vi "Gets_data.vi"(0 "object in":refnum<class "212format_work.lvclass">, 5 "error in (no error)":errorcluster) -> (14 "object out":refnum<class "212format_work.lvclass">, 15 "data":T1={"选择发送的参数"="", "插值后的数组元素"={"PH"=[], "CODCr"=[], "氨氮"=[], "CODMn"=[], "总氮"=[], "总磷"=[], "电导率"=[], "水温"=[], "DO"=[], "浊度"=[], "叶绿素"=[], "藻密度"=[], "铜"=[], "盐度"=[], "水位"=[], "流速"=[], "瞬时流量"=[], "累积流量"=[], "亚硝酸盐"=[], "硫化物"=[], "ORP"=[], "铅"=[], "镉"=[], "锌"=[], "镍"=[], "锰"=[], "汞"=[], "气温"=[], "气压"=[], "风速"=[], "风向"=[], "盐度 2"=[], "磷酸盐"=[], "硝氮"=[], "氟化物"=[], "挥发酚"=[], "氯化物"=[]}, "register values"=[], "columns输出"=[], "环境参数"=[], "仪器编码"="", "实时数据发送间隔"=0, "实时数据参数"="水样测试", "参数系数簇"={"CODMn"=0.0, "CODCr"=0.0, "DO"=0.0, "铜"=0.0, "PH"=0.0, "氨氮"=0.0, "比电导率"=0.0, "水温"=0.0, "COD"=0.0, "浊度"=0.0, "总氮"=0.0, "总磷"=0.0, "叶绿素a"=0.0, "藻密度"=0.0, "水位"=0.0, "流速"=0.0, "瞬时流量"=0.0, "累积流量"=0.0, "亚硝酸盐"=0.0, "硫化物"=0.0, "ORP"=0.0, "铅"=0.0, "镉"=0.0, "锌"=0.0, "镍"=0.0, "锰"=0.0, "汞"=0.0, "气温"=0.0, "气压"=0.0, "风速"=0.0, "风向"=0.0, "盐度"=0.0, "磷酸盐"=0.0, "硝氮"=0.0, "氟化物"=0.0, "挥发酚"=0.0, "氯化物"=0.0}, "因子编码簇"={"CODMn"="", "CODCr"="", "DO"="", "铜"="", "PH"="", "氨氮"="", "比电导率"="", "水温"="", "COD"="", "浊度"="", "总氮"="", "总磷"="", "叶绿素a"="", "藻密度"="", "水位"="", "流速"="", "瞬时流量"="", "累积流量"="", "亚硝酸盐"="", "硫化物"="", "ORP"="", "铅"="", "镉"="", "锌"="", "镍"="", "锰"="", "汞"="", "气温"="", "气压"="", "风速"="", "风向"="", "盐度"="", "磷酸盐"="", "硝氮"="", "氟化物"="", "挥发酚"="", "氯化物"=""}, "小时数据发送次数"=0, "读取试剂余量的值"=[], "参数编码"="", "数据数组大小"=0, "总包数"=0, "当前包号"=0, "columns"=[], "剖面多参数"=[], "分包标准"=3}, 19 "error out":errorcluster)   [LabVIEW 2016, in "212format_work.lvclass"]
uses:
  212format_work.lvclass
  212format_work.lvclass/212format_work.ctl
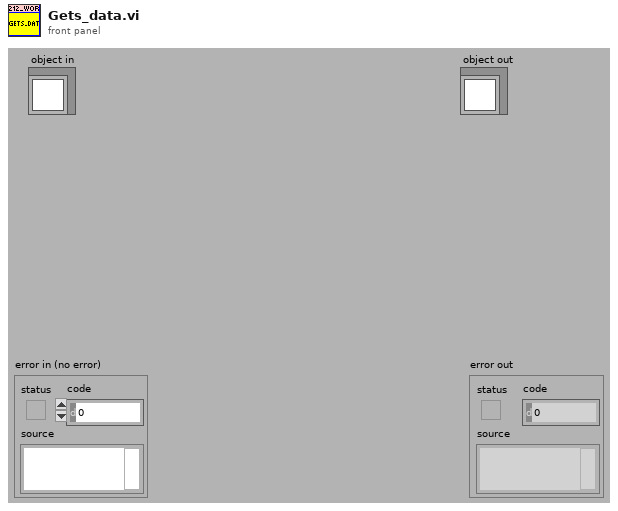
[diagram p1: front panel]
types:
  T1 = typedef "212format_work.lvclass/data控件.ctl" = cluster{"选择发送的参数":string, "插值后的数组元素":cluster{"PH":string[][], "CODCr":string[][], "氨氮":string[][], "CODMn":string[][], "总氮":string[][], "总磷":string[][], "电导率":string[][], "水温":string[][], "DO":string[][], "浊度":string[][], "叶绿素":string[][], "藻密度":string[][], "铜":string[][], "盐度":string[][], "水位":string[][], "流速":string[][], "瞬时流量":string[][], "累积流量":string[][], "亚硝酸盐":string[][], "硫化物":string[][], "ORP":string[][], "铅":string[][], "镉":string[][], "锌":string[][], "镍":string[][], "锰":string[][], "汞":string[][], "气温":string[][], "气压":string[][], "风速":string[][], "风向":string[][], "盐度 2":string[][], "磷酸盐":string[][], "硝氮":string[][], "氟化物":string[][], "挥发酚":string[][], "氯化物":string[][]}, "register values":u16[], "columns输出":string[], "环境参数":string[][], "仪器编码":string, "实时数据发送间隔":u32, "实时数据参数":string, "参数系数簇":cluster{"CODMn":dbl, "CODCr":dbl, "DO":dbl, "铜":dbl, "PH":dbl, "氨氮":dbl, "比电导率":dbl, "水温":dbl, "COD":dbl, "浊度":dbl, "总氮":dbl, "总磷":dbl, "叶绿素a":dbl, "藻密度":dbl, "水位":dbl, "流速":dbl, "瞬时流量":dbl, "累积流量":dbl, "亚硝酸盐":dbl, "硫化物":dbl, "ORP":dbl, "铅":dbl, "镉":dbl, "锌":dbl, "镍":dbl, "锰":dbl, "汞":dbl, "气温":dbl, "气压":dbl, "风速":dbl, "风向":dbl, "盐度":dbl, "磷酸盐":dbl, "硝氮":dbl, "氟化物":dbl, "挥发酚":dbl, "氯化物":dbl}, "因子编码簇":cluster{"CODMn":string, "CODCr":string, "DO":string, "铜":string, "PH":string, "氨氮":string, "比电导率":string, "水温":string, "COD":string, "浊度":string, "总氮":string, "总磷":string, "叶绿素a":string, "藻密度":string, "水位":string, "流速":string, "瞬时流量":string, "累积流量":string, "亚硝酸盐":string, "硫化物":string, "ORP":string, "铅":string, "镉":string, "锌":string, "镍":string, "锰":string, "汞":string, "气温":string, "气压":string, "风速":string, "风向":string, "盐度":string, "磷酸盐":string, "硝氮":string, "氟化物":string, "挥发酚":string, "氯化物":string}, "小时数据发送次数":i32, "读取试剂余量的值":u16[], "参数编码":string, "数据数组大小":i32, "总包数":i32, "当前包号":i32, "columns":string[], "剖面多参数":string[][], "分包标准":i32}
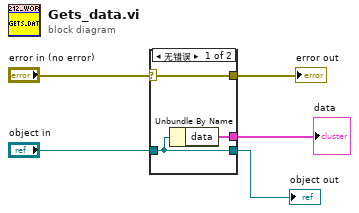
[diagram p0: block diagram]
diagram:
  n1 = case shown="无错误" "error in (no error)" {
    selector: "error in (no error)" -> [w7 w10]
    tunnel: [w7 w10] -> w4
    tunnel: [w6 w9] -> w2
    tunnel: "object in" -> [w6 w9]
    tunnel: [w8 _] -> w1
    frame No Error {
      n2 = Unbundle By Name(w6) -> ("data"=w8:T1)
    }
    frame Error {
    }
  }
  "error out" <- w4
  "object out" <- w2
  "data" <- w1
